vi "UnpackFieldsFromAny.vi"(8 "error in":errorcluster, 11 "Any":T1) -> (0 "error out":errorcluster, 3 "Fields Ref Out":T2)   [LabVIEW 2019, in "grpc-lvsupport.lvlib"]
uses:
  grpc-lvsupport.lvlib
  grpcId.ctl
  Any.ctl
  <vilib>/Utility/error.llb/Error Cluster From Error Code.vi
  <resource>/labview_grpc_server.dll
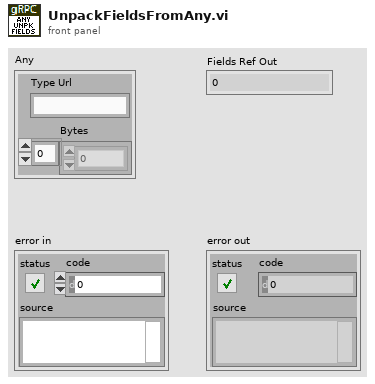
[diagram p1: front panel]
types:
  T1 = typedef "grpc-lvsupport.lvlib/Any.ctl" = cluster{"Type Url":string, "Bytes":u8[]}
  T2 = typedef "grpc-lvsupport.lvlib/grpcId.ctl" = u64
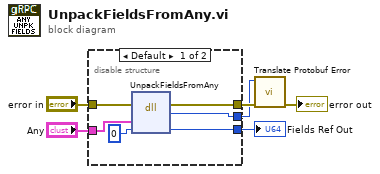
[diagram p0: block diagram]
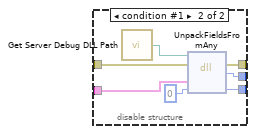
[diagram p2: hidden frame]
diagram:
  n1 = disable-structure shown="Default" {
    disable-tunnel: "error in" -> [w12 w19]
    disable-tunnel: [w11 w18] -> w5
    disable-tunnel: [w10 w16] -> w4
    disable-tunnel: "Any" -> [w9 w15]
    disable-tunnel: [w8 w14] -> w1
    frame condition #0 (active) {
      n2 = dll-call lib="C:/Program Files (x86)/National Instruments/LabVIEW 2024/resource/labview_grpc_server.*" fn="UnpackFieldsFromAny"(error in=w12, "any"=w9, "elementRef"=u64 0) -> (error out=w11:errorcluster, "return type"=w8:i32, "elementRef"=w10:u64)  [unwired: 3 in, 1 out]
    }
    frame condition #1 {
      n3 = call "Get Server Debug DLL Path.vi"() -> ("DLL Path"=w17:path)
      n4 = dll-call lib="?" fn="UnpackFieldsFromAny"(path in=w17, error in=w19, "any"=w15, "elementRef"=u64 0) -> (error out=w18:errorcluster, "return type"=w14:i32, "elementRef"=w16:u64)  [unwired: 2 in, 1 out]
    }
  }
  "Fields Ref Out" <- w4
  n5 = call "Translate Protobuf Error.vi"("error in"=w5, "Error Code"=w1) -> ("error out"=→"error out":errorcluster)  [unwired: 9 in]
